vi "TCP Close DAQ STATUS Connection.vi"(8 "error in (no error)":errorcluster) -> (0 "error out":errorcluster)   [LabVIEW 2015]
uses:
  DAQ Engine VIs/PXI Globals.vi
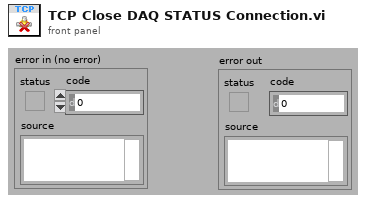
[diagram p1: front panel]
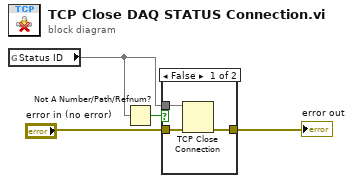
[diagram p0: block diagram]
diagram:
  n1 = global read "PXI Globals.vi" "Status ID"() -> (w3)
  n2 = Not A Number/Path/Refnum?(number/path/refnum=w3) -> (NaN/Path/Refnum?=w2:bool)
  n3 = case shown="False" w2 {
    tunnel: [w7 w8] -> w1
    tunnel: "error in (no error)" -> [w6 w8]
    tunnel: w3 -> [w5 _]
    frame False {
      n4 = TCP Close Connection(connection ID=w5, error in (no error)=w6) -> (error out=w7:errorcluster)  [unwired: 1 in, 1 out]
    }
    frame True {
    }
  }
  "error out" <- w1
